vi "Get Logic Status (single).vi"(8 "error in (no error)":errorcluster, 10 "Pin # (1-based)":u8, 11 "LogicIO in":refnum<class "LogicIO.lvclass">) -> (0 "error out":errorcluster, 2 "logic status":bool, 3 "LogicIO out":refnum<class "LogicIO.lvclass">)   [LabVIEW 2016, in "Hardware.lvlib" / "LogicIO.lvlib" / "LogicIO.lvclass"]
uses:
  <userlib>/Common Components/Hardware/LogicIO/LogicIO/LogicIO.lvclass
  <vilib>/Utility/error.llb/Error Cluster From Error Code.vi
  <vilib>/ErrorRing/Error Ring.xnode
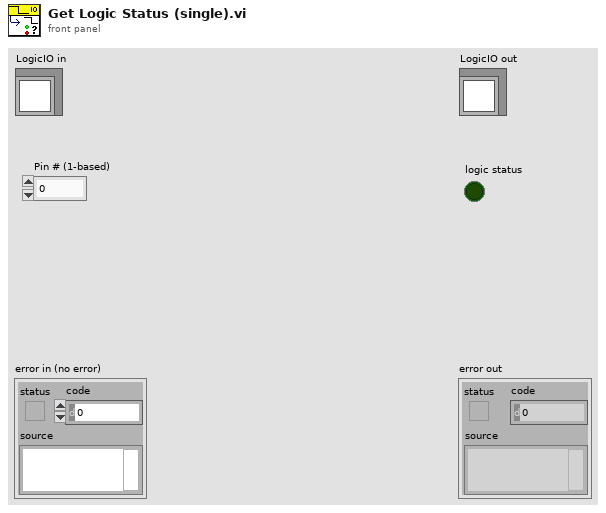
[diagram p1: front panel]
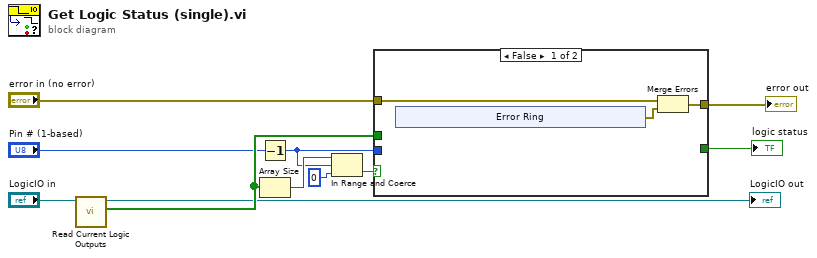
[diagram p0: block diagram]
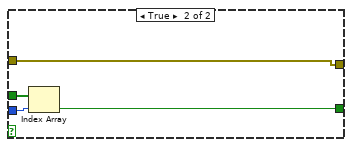
[diagram p2: hidden frame]
diagram:
  n1 = call <userlib>:"Read Current Logic Outputs.vi"("LogicIO in"="LogicIO in") -> ("Current Logic Outputs"=w8:bool[], "LogicIO out"=→"LogicIO out":refnum<class "LogicIO.lvclass">)  [unwired: 9 in]
  n2 = Decrement(x="Pin # (1-based)") -> (x-1=w1:u8)
  n3 = Array Size(array=w8) -> (size(s)=w4:i32)
  n4 = In Range and Coerce(upper limit=w4, x=w1, lower limit=0) -> (In Range?=w2:bool)  [unwired: 1 out]
  n5 = case shown="False" w2 {
    tunnel: w8 -> [_ w22]
    tunnel: w1 -> [_ w21]
    tunnel: [_ w20] -> w11
    tunnel: "error in (no error)" -> [w12 w19]
    tunnel: [w13 w19] -> w9
    frame False {
      n6 = xnode "Error Ring"() -> ("error out"=w14:errorcluster)
      n7 = Merge Errors(w12, w14) -> (w13:errorcluster)
    }
    frame True {
      n8 = Index Array(array=w22, index=w21) -> (element=w20:bool)
    }
  }
  "error out" <- w9
  "logic status" <- w11
